vi "max_min_range.vi"(2 "Z Min/Max":T1) -> (7 "Range":sgl)   [LabVIEW 2020, in "3DPC_SurfacePlot.xctl"]
uses:
  <vilib>/Native 3D Graph/xcontrol/3DPC_SurfacePlot.xctl
  <vilib>/Native 3D Graph/typedefs/min_max.ctl
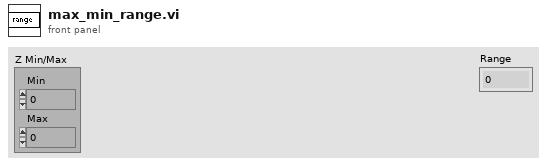
[diagram p1: front panel]
types:
  T1 = typedef "3DPC_SurfacePlot.xctl/min_max.ctl" = cluster{"Min":sgl, "Max":sgl}
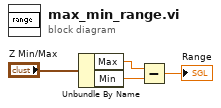
[diagram p0: block diagram]
diagram:
  n1 = Unbundle By Name("Z Min/Max") -> ("Max"=w2:sgl, "Min"=w3:sgl)
  n2 = Subtract(x=w2, y=w3) -> (x-y=→"Range":sgl)
